vi "题目1.vi"() -> ()   [LabVIEW 2017]
panel:
  out "波形图 7":cluster{i32, i32, cluster{dbl[]}[]}(graph)
  out "波形图 6":cluster{i32, i32, dbl[][]}(graph)
  out "波形图 5":cluster{i32, i32, dbl[]}[](graph)
  out "波形图 4":cluster{i32, i32, dbl[]}(graph)
  out "波形图 3":cluster{dbl[]}[](graph)
  out "波形图 2":dbl[][](graph)
  out "波形图":dbl[](graph)
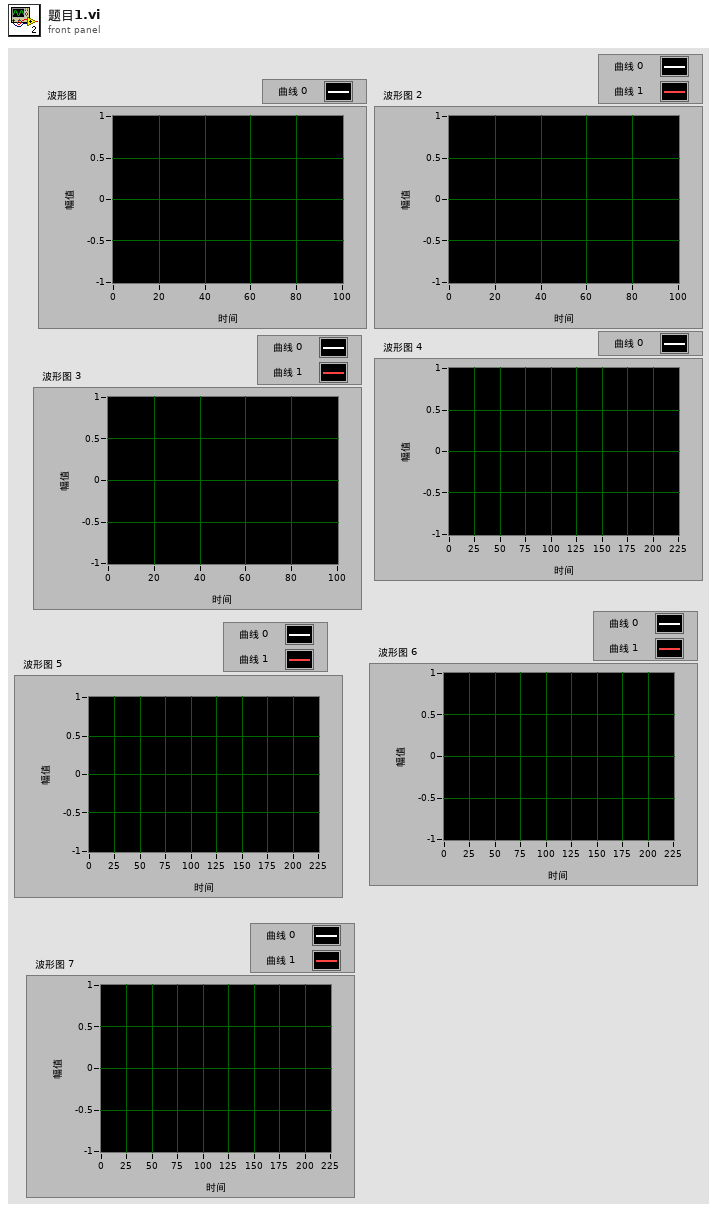
[diagram p1: front panel]
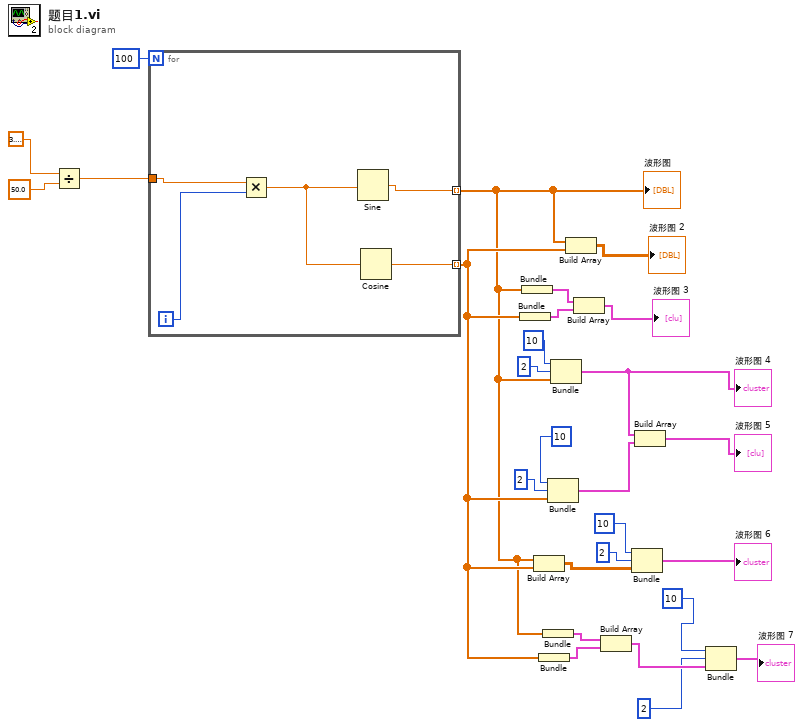
[diagram p0: block diagram]
diagram:
  n1 = Divide(x=3.141592653589793, y=50.0) -> (x/y=w25:dbl)
  n2 = for {
    N: 100 -> [_]
    tunnel: w25 -> [w32]
    tunnel: [w30] -> w7 mode=indexing
    tunnel: [w28] -> w8 mode=indexing
    i -> [w31]
    n3 = Multiply(x=w32, y=w31) -> (x*y=w29:dbl)
    n4 = Sine(x=w29) -> (sin(x)=w30:dbl)
    n5 = Cosine(x=w29) -> (cos(x)=w28:dbl)
  }
  "波形图" <- w7
  n6 = Bundle(w8) -> (w21:cluster{dbl[]})  [unwired: 1 in]
  n7 = Bundle(w7) -> (w22:cluster{dbl[]})  [unwired: 1 in]
  n8 = Build Array(w7, w8) -> (w12:dbl[][])
  n9 = Bundle(w8) -> (w5:cluster{dbl[]})  [unwired: 1 in]
  n10 = Bundle(w7) -> (w6:cluster{dbl[]})  [unwired: 1 in]
  n11 = Bundle(10, 2, w8) -> (w14:cluster{i32, i32, dbl[]})  [unwired: 1 in]
  n12 = Bundle(10, 2, w7) -> (w15:cluster{i32, i32, dbl[]})  [unwired: 1 in]
  "波形图 4" <- w15
  n13 = Build Array(w7, w8) -> (→"波形图 2":dbl[][])
  n14 = Build Array(w22, w21) -> (→"波形图 3":cluster{dbl[]}[])
  n15 = Build Array(w6, w5) -> (w4:cluster{dbl[]}[])
  n16 = Bundle(10, 2, w12) -> (→"波形图 6":cluster{i32, i32, dbl[][]})  [unwired: 1 in]
  n17 = Build Array(w15, w14) -> (→"波形图 5":cluster{i32, i32, dbl[]}[])
  n18 = Bundle(10, 2, w4) -> (→"波形图 7":cluster{i32, i32, cluster{dbl[]}[]})  [unwired: 1 in]
